vi "Get Project Items.vi"(7 "Calling VI Ref":refnum<vi>, 8 "error in (no error)":errorcluster, 11 "Path":path) -> (0 "error out":errorcluster, 2 "Cancelled?":bool, 3 "Items Data":refnum<class "Item.lvclass">[](array[class]))   [LabVIEW 2020, in "VI Properties Editor.lvlib"]
doc: "Initializes class data for all items contained within the project identified by <B>Path</B>."
uses:
  VI Properties Editor.lvlib
  Classes/Item/Item.lvclass
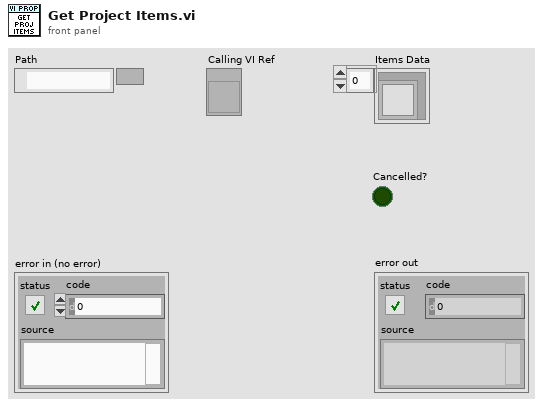
[diagram p1: front panel]
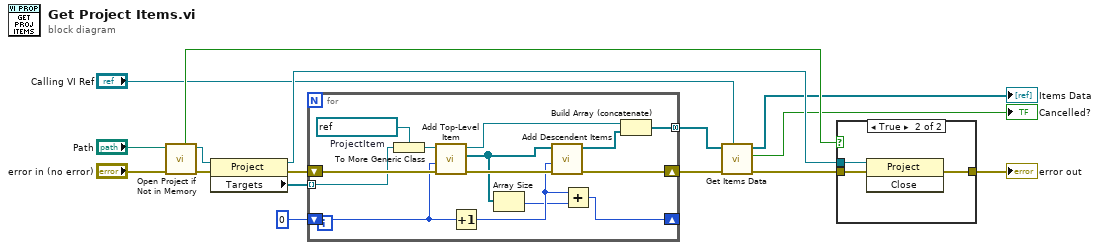
[diagram p0: block diagram]
diagram:
  n1 = call "Open Project if Not in Memory.vi"("error in (no error)"="error in (no error)", "Path"="Path") -> ("error out"=w12:errorcluster, "Project Ref"=w10:refnum<vi>, "Opened?"=w7:bool)  [unwired: 7 in]
  n2 = property class="Project"(reference=w10, error in=w12) -> (reference out=w16:refnum<vi>, error out=w15:errorcluster, "Targets"=w14:refnum<vi>[])
  n3 = for {
    tunnel: w14 -> [w22] mode=indexing
    shift-right: [w28] -> w13
    shift-left: w15 -> [w30]
    shift-right: [w24] -> _
    shift-left: 0 -> [w27]
    tunnel: [w19] -> w3 mode=concatenating
    w17 = refnum<vi> refnum  # ProjectItem
    n4 = To More Generic Class(target class=w17, reference=w22) -> (generic class reference=w18:refnum<vi>)
    n5 = call "Add Top-Level Item.vi"("error in (no error)"=w30, "Order"=w27, "ProjectItem Ref"=w18) -> ("error out"=w29:errorcluster, "Descendents Refs"=w23:refnum<vi>[], "Item"=w21:refnum<class "Item.lvclass">)  [unwired: 6 in]
    n6 = Increment(x=w27) -> (x+1=w26:i32)
    n7 = Array Size(array=w23) -> (size(s)=w25:i32)
    n8 = call "Add Descendent Items.vi"("error in (no error)"=w29, "Order"=w26, "Descendents Refs"=w23) -> ("error out"=w28:errorcluster, "Items"=w20:refnum<class "Item.lvclass">[])  [unwired: 7 in]
    n9 = Add(x=w26, y=w25) -> (x+y=w24:i32)
    n10 = Build Array (concatenate)(w21, w20) -> (w19:refnum<class "Item.lvclass">[])
  }
  n11 = call "Get Items Data.vi"("Calling VI Ref"="Calling VI Ref", "error in (no error)"=w13, "Items"=w3) -> ("error out"=w6:errorcluster, "Cancelled?"=→"Cancelled?":bool, "Items out"=→"Items Data":refnum<class "Item.lvclass">[])  [unwired: 6 in]
  n12 = case shown="True" w7 {
    tunnel: w6 -> [w31 w34]
    tunnel: w16 -> [_ w33]
    tunnel: [w31 w32] -> w8
    frame False {
    }
    frame True {
      n13 = invoke class="Project" method="Close"(reference=w33, error in=w34) -> (error out=w32:errorcluster)  [unwired: 1 in, 2 out]
    }
  }
  "error out" <- w8
